vi "ExecuteMenu.vi"(8 "ErrorIn":errorcluster, 10 "ItemPath":string, 11 "MasterGUIIn":refnum<class "MasterGUI.lvclass">) -> (0 "ErrorOut":errorcluster, 3 "MasterGUIOut":refnum<class "MasterGUI.lvclass">)   [LabVIEW 2021, in "MasterGUI.lvclass"]
uses:
  MasterGUI.lvclass
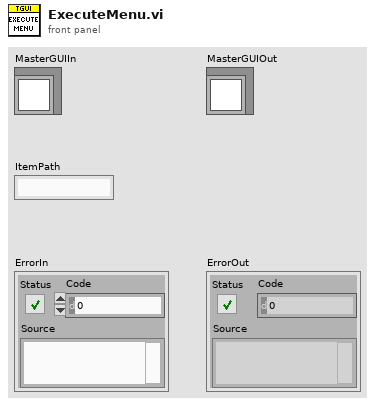
[diagram p1: front panel]
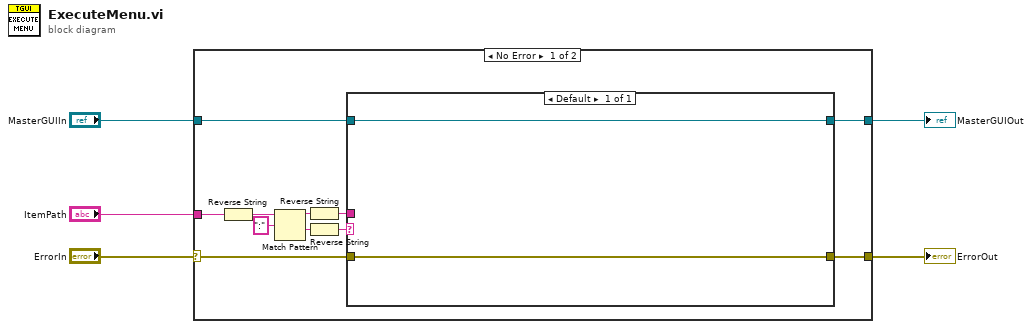
[diagram p0: block diagram]
diagram:
  n1 = case shown="No Error" "ErrorIn" {
    selector: "ErrorIn" -> [w15 w20]
    tunnel: [w14 w19] -> w3
    tunnel: "MasterGUIIn" -> [w13 w19]
    tunnel: [w16 w20] -> w5
    tunnel: "ItemPath" -> [w6 _]
    frame No Error {
      n2 = Reverse String(1:w6) -> (0:w10:string)
      n3 = Match Pattern(string=w10, regular expression=":") -> (before substring=w8:string, after substring=w9:string)  [unwired: 1 in, 2 out]
      n4 = Reverse String(1:w8) -> (0:w11:string)
      n5 = Reverse String(1:w9) -> (0:w12:string)
      n6 = case shown="Default" w12 {
        tunnel: w11 -> [_]
        tunnel: [w18] -> w16
        tunnel: w15 -> [w18]
        tunnel: [w17] -> w14
        tunnel: w13 -> [w17]
        frame Default {
        }
      }
    }
    frame Error {
    }
  }
  "MasterGUIOut" <- w3
  "ErrorOut" <- w5
